vi "Add Caption and Table.vi"(0 "PDF Report IN":refnum<class "PDF Report Class.lvclass">, 2 "Caption?":bool, 5 "Paragraph Refnum":refnum<k24>, 7 "PdfPTable":refnum<k24>, 11 "error in (no error)":errorcluster) -> (4 "PDF Report OUT":refnum<class "PDF Report Class.lvclass">, 15 "error out":errorcluster)   [LabVIEW 2019, in "Exaprom PDF.lvlib"]
doc: "Version 2.0\nDeveloped by Jean-Marc Simard\nCopyright © 2012, Exaprom Inc.\nAll rights reserved.\nLicense: BSD\n\nWith iTextSharp 4.1.6 (http://itextsharp.sourceforge.net)\nunder Mozilla Public License Version 1.1\n(http://www.mozilla.org/MPL/MPL-1.1.html)"
uses:
  LV Class/PDF Report Class/PDF Report Class.lvclass
  C:/work/niobrara_lv/labview pdf writer fixing/DLL/itextsharp.dll
  DLL/itextsharp.dll
  Exaprom PDF.lvlib
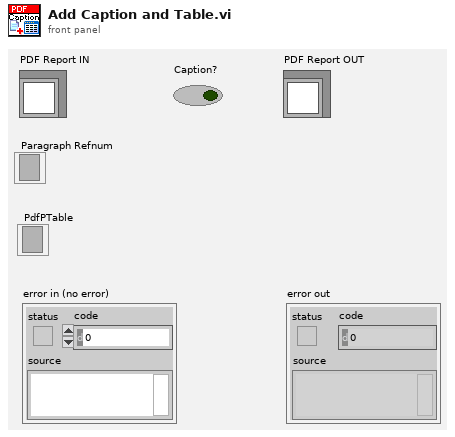
[diagram p1: front panel]
types:
  T1 = typedef "Exaprom PDF.lvlib/Captions.ctl" = cluster{"Figure":T2, "Table":T2, "Font":T3}
  T2 = typedef "Exaprom PDF.lvlib/Image or Table Caption.ctl" = cluster{"Caption":string, "Separator":string, "Position":enum16{"Above", "Below"}}
  T3 = typedef "Exaprom PDF.lvlib/Font complete cluster.ctl" = cluster{"Name":string, "Size":T4, "Color":T5, "Style":cluster{"Bold":bool, "Italic":bool, "Underline":bool, "Strikeout":bool}, "Type":T6}
  T4 = typedef "Exaprom PDF.lvlib/Font size.ctl" = sgl
  T5 = typedef "Exaprom PDF.lvlib/Font color.ctl" = u32
  T6 = typedef "Exaprom PDF.lvlib/Type and encoding.ctl" = cluster{"Type&direction":T7, "Embedded":bool, "Encoding":string}
  T7 = typedef "Exaprom PDF.lvlib/Type and run direction.ctl" = enum16{"Select", "ASCII", "UTF-16", "UTF-16 (default)", "UTF-16 (LTR)", "UTF-16 (RTL)"}
  T8 = cluster{"Captions":T1, "Image counter":u16, "Table counter":u16}
  T9 = cluster{"HorizontalAlignment":i32, "SpacingBefore":sgl, "SpacingAfter":sgl}
  T10 = cluster{"HorizontalAlignment":i32, "SpacingAfter":sgl, "SpacingAfter":sgl}
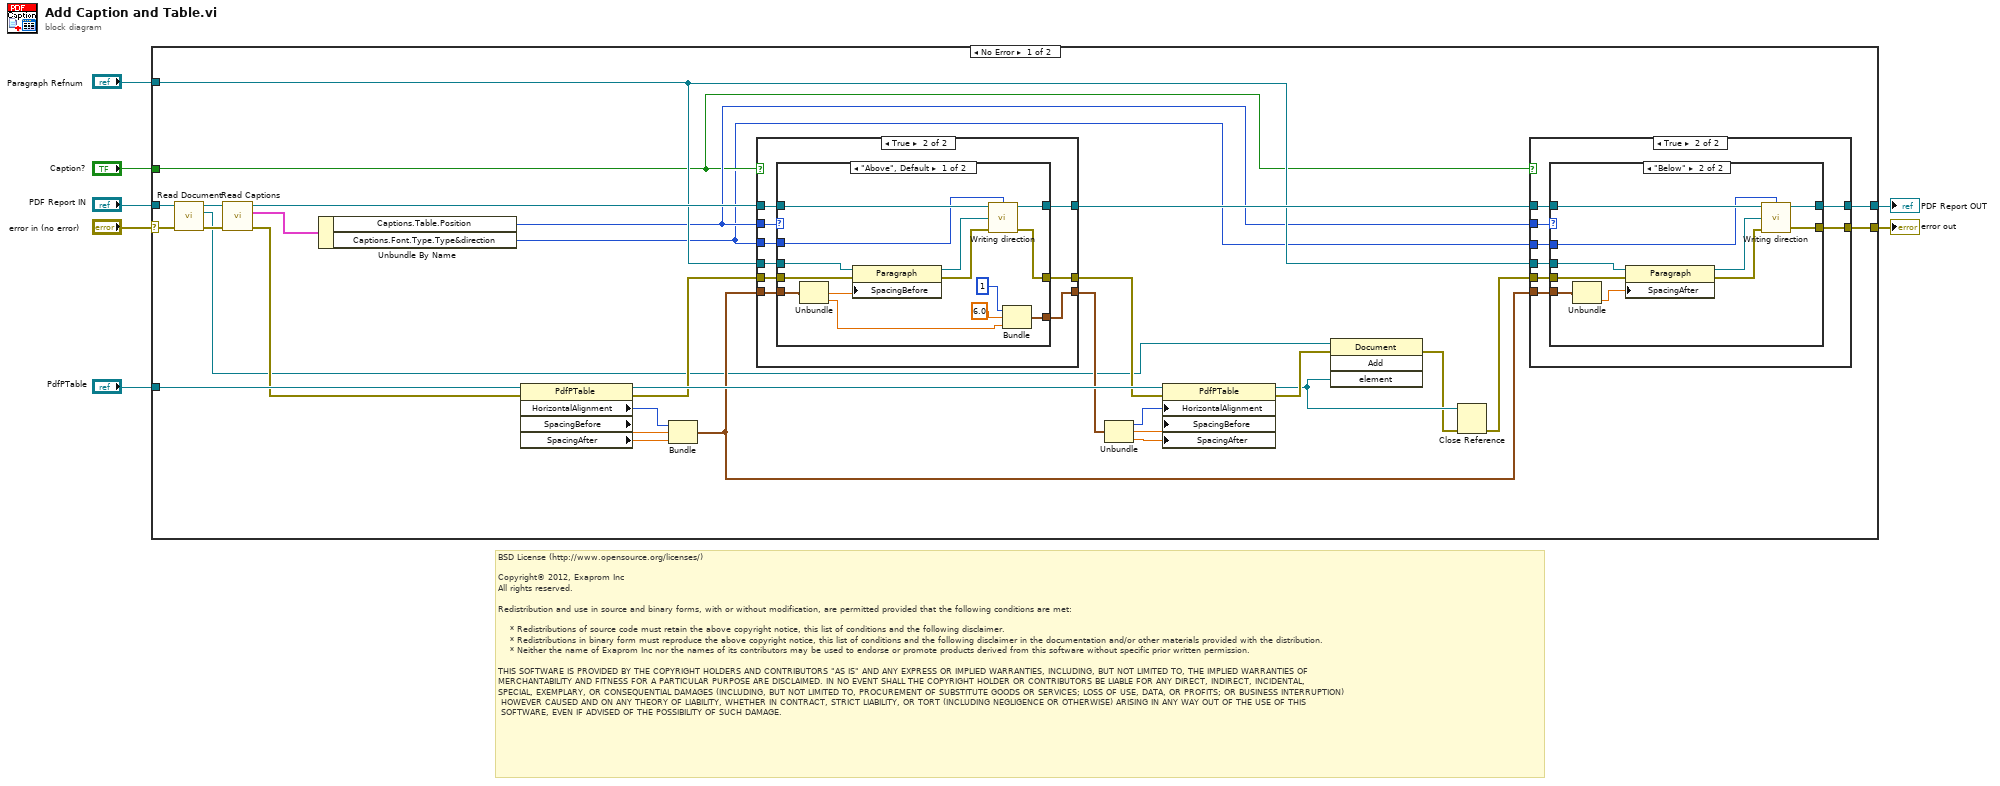
[diagram p0: block diagram]
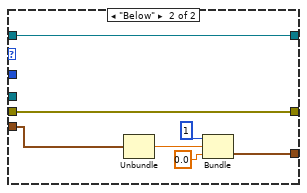
[diagram p5: hidden frame]
diagram:
  # "BSD License (http://www.opensource.org/licenses/)\n\nCopyright© 2012, Exaprom Inc\nAll rights reserved.\n\nRedistribution and use in source and binary forms, with or without modification, are permitted provided that the following conditions are met:\n\n    * Redistributions of source code must retain the above copyright notice, this list of conditions and the following disclaimer.\n    * Redistributions in binary form must reproduce the above copyright notice, this list of conditions and the following disclaimer in the documentation and/or other materials provided with the distribution.\n    * Neither the name of Exaprom Inc nor the names of its contributors may be used to endorse or promote products derived from this software without specific prior written permission.\n\nTHIS SOFTWARE IS PROVIDED BY THE COPYRIGHT HOLDERS AND CONTRIBUTORS \"AS IS\" AND ANY EXPRESS OR IMPLIED WARRANTIES, INCLUDING, BUT NOT LIMITED TO, THE IMPLIED WARRANTIES OF \nMERCHANTABILITY AND FITNESS FOR A PARTICULAR PURPOSE ARE DISCLAIMED. IN NO EVENT SHALL THE COPYRIGHT HOLDER OR CONTRIBUTORS BE LIABLE FOR ANY DIRECT, INDIRECT, INCIDENTAL,\nSPECIAL, EXEMPLARY, OR CONSEQUENTIAL DAMAGES (INCLUDING, BUT NOT LIMITED TO, PROCUREMENT OF SUBSTITUTE GOODS OR SERVICES; LOSS OF USE, DATA, OR PROFITS; OR BUSINESS INTERRUPTION)\n HOWEVER CAUSED AND ON ANY THEORY OF LIABILITY, WHETHER IN CONTRACT, STRICT LIABILITY, OR TORT (INCLUDING NEGLIGENCE OR OTHERWISE) ARISING IN ANY WAY OUT OF THE USE OF THIS\n SOFTWARE, EVEN IF ADVISED OF THE POSSIBILITY OF SUCH DAMAGE."
  n1 = case shown="No Error" "error in (no error)" {
    selector: "error in (no error)" -> [w23 w95]
    tunnel: "PDF Report IN" -> [w27 w94]
    tunnel: [w11 w94] -> w6
    tunnel: [w10 w95] -> w5
    tunnel: "PdfPTable" -> [w28 _]
    tunnel: "Caption?" -> [w12 _]
    tunnel: "Paragraph Refnum" -> [w14 _]
    frame No Error {
      n2 = call-dynamic "Read Document.vi"("error in (no error)"=w23, "PDF Report Class in"=w27) -> ("error out"=w25:errorcluster, "Document"=w9:refnum<k24>, "PDF Report Class out"=w24:refnum<class "PDF Report Class.lvclass">)  [unwired: 7 in]
      n3 = call-dynamic "Read Captions.vi"("error in (no error)"=w25, "PDF Report Class in"=w24) -> ("error out"=w22:errorcluster, "Captions and counters"=w26:T8, "PDF Report Class out"=w20:refnum<class "PDF Report Class.lvclass">)  [unwired: 7 in]
      n4 = Unbundle By Name(w26) -> ("Captions.Table.Position"=w13:enum16{"Above", "Below"}, "Captions.Font.Type.Type&direction"=w8:T7)
      n5 = property class="PdfPTable"(reference=w28, error in=w22) -> (reference out=w38:refnum<k24>, error out=w21:errorcluster, "HorizontalAlignment"=w35:i32, "SpacingBefore"=w36:sgl, "SpacingAfter"=w37:sgl)
      n6 = Bundle("HorizontalAlignment"=w35, "SpacingBefore"=w36, "SpacingAfter"=w37) -> (w15:T9)  [unwired: 1 out]
      n7 = case shown="True" w12 {
        tunnel: w21 -> [w63 w72]
        tunnel: [w63 w71] -> w18
        tunnel: w13 -> [_ w70]
        tunnel: w14 -> [_ w69]
        tunnel: w20 -> [w62 w68]
        tunnel: [w62 w67] -> w17
        tunnel: w8 -> [_ w66]
        tunnel: w15 -> [w61 w65]
        tunnel: [w61 w64] -> w19
        frame False {
        }
        frame True {
          n8 = case shown="\"Above\", Default" w70 {
            tunnel: w69 -> [w78 _]
            tunnel: w72 -> [w80 w93]
            tunnel: [w84 w93] -> w71
            tunnel: w68 -> [w86 w92]
            tunnel: [w85 w92] -> w67
            tunnel: w66 -> [w83 _]
            tunnel: w65 -> [w81 w87]
            tunnel: [w74 w88] -> w64
            frame "Above", Default {
              n9 = Unbundle(w81) -> ("SpacingBefore"=w82:sgl, "SpacingAfter"=w75:sgl)  [unwired: 1 out]
              n10 = property class="Paragraph"(reference=w78, error in=w80, "SpacingBefore"=w82) -> (reference out=w73:refnum<k24>, error out=w79:errorcluster)
              n11 = call "Writing direction.vi"("PDF Report IN"=w86, "Text type"=w83, "Paragraph refnum"=w73, "error in (no error)"=w79) -> ("PDF Report OUT"=w85:refnum<class "PDF Report Class.lvclass">, "error out"=w84:errorcluster)  [unwired: 10 in]
              n12 = Bundle("HorizontalAlignment"=1, "SpacingAfter"=sgl 6.0, "SpacingAfter"=w75) -> (w74:T10)  [unwired: 1 out]
            }
            frame "Below" {
              n13 = Unbundle(w87) -> ("SpacingBefore"=w90:sgl)  [unwired: 2 out]
              n14 = Bundle("HorizontalAlignment"=1, "SpacingBefore"=w90, "SpacingAfter"=sgl 0.0) -> (w88:T9)  [unwired: 1 out]
            }
          }
        }
      }
      n15 = Unbundle(w19) -> ("HorizontalAlignment"=w32:i32, "SpacingBefore"=w33:sgl, "SpacingAfter"=w34:sgl)
      n16 = property class="PdfPTable"(reference=w38, error in=w18, "HorizontalAlignment"=w32, "SpacingBefore"=w33, "SpacingAfter"=w34) -> (reference out=w30:refnum<k24>, error out=w31:errorcluster)
      n17 = invoke class="Document" method="Add"(reference=w9, error in=w31, "element"=w30) -> (error out=w29:errorcluster)  [unwired: 1 in, 3 out]
      n18 = Close Reference(reference=w30, error in (no error)=w29) -> (error out=w16:errorcluster)
      n19 = case shown="True" w12 {
        tunnel: w16 -> [w40 w48]
        tunnel: [w40 w47] -> w10
        tunnel: w13 -> [_ w46]
        tunnel: w14 -> [_ w45]
        tunnel: w17 -> [w39 w44]
        tunnel: [w39 w43] -> w11
        tunnel: w8 -> [_ w42]
        tunnel: w15 -> [_ w41]
        frame False {
        }
        frame True {
          n20 = case shown="\"Below\"" w46 {
            tunnel: w45 -> [_ w53]
            tunnel: w48 -> [w50 w55]
            tunnel: [w50 w58] -> w47
            tunnel: w44 -> [w49 w60]
            tunnel: [w49 w59] -> w43
            tunnel: w42 -> [_ w57]
            tunnel: w41 -> [_ w56]
            frame "Above", Default {
            }
            frame "Below" {
              n21 = Unbundle(w56) -> ("SpacingAfter"=w52:sgl)  [unwired: 2 out]
              n22 = property class="Paragraph"(reference=w53, error in=w55, "SpacingAfter"=w52) -> (reference out=w51:refnum<k24>, error out=w54:errorcluster)
              n23 = call "Writing direction.vi"("PDF Report IN"=w60, "Text type"=w57, "Paragraph refnum"=w51, "error in (no error)"=w54) -> ("PDF Report OUT"=w59:refnum<class "PDF Report Class.lvclass">, "error out"=w58:errorcluster)  [unwired: 10 in]
            }
          }
        }
      }
    }
    frame Error {
    }
  }
  "PDF Report OUT" <- w6
  "error out" <- w5
